vi "Size.vi"(8 "error in (no error)":errorcluster, 11 "Cluster Array in":refnum<class "Cluster Array.lvclass">) -> (0 "error out":errorcluster, 2 "Size":i32, 3 "Cluster Array out":refnum<class "Cluster Array.lvclass">)   [LabVIEW 2020, in "Data.lvlib" / "Cluster Array.lvclass"]
doc: "Return the size of the generic data element."
uses:
  Cluster Array.lvclass
  Cluster Array.lvclass/Cluster Array.ctl
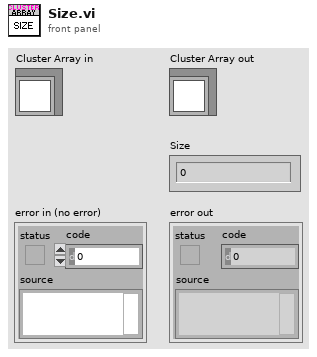
[diagram p1: front panel]
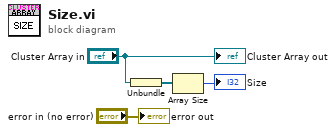
[diagram p0: block diagram]
diagram:
  n1 = Unbundle("Cluster Array in") -> (w2:refnum<class "Cluster.lvclass">[])
  n2 = Array Size(array=w2) -> (size(s)=→"Size":i32)
  "error out" <- "error in (no error)"
  "Cluster Array out" <- "Cluster Array in"
